vi "Create Test Class.vi"(8 "error in (no error)":errorcluster, 11 "Test Double Factory in":refnum<class "Test Double Factory.lvclass">) -> (0 "error out":errorcluster, 3 "Test Double Factory out":refnum<class "Test Double Factory.lvclass">)   [LabVIEW 2020, in "Test Double Factory.lvclass"]
uses:
  Test Double Factory.lvclass
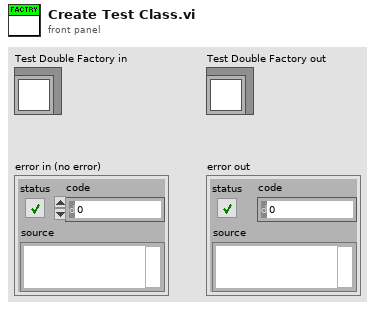
[diagram p1: front panel]
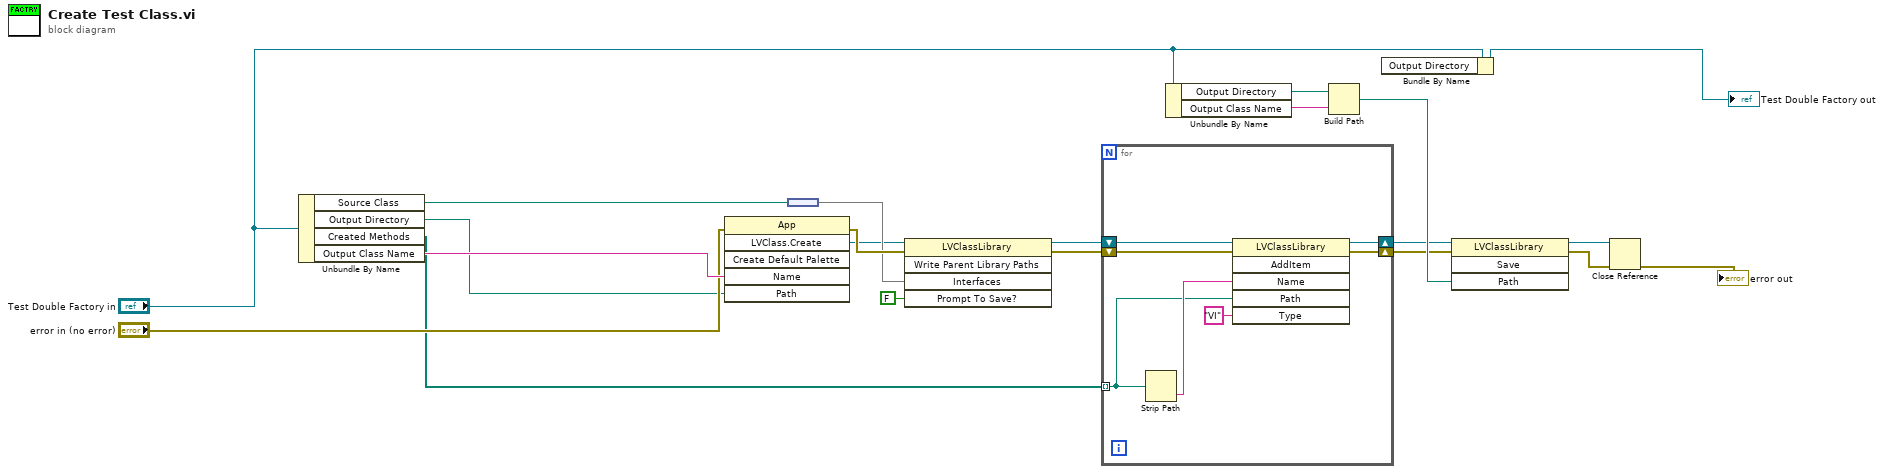
[diagram p0: block diagram]
diagram:
  n1 = Unbundle By Name("Test Double Factory in") -> ("Source Class"=w6:path, "Output Directory"=w5:path, "Created Methods"=w9:path[], "Output Class Name"=w19:string)
  n2 = invoke class="App" method="LVClass.Create"(error in="error in (no error)", "Name"=w19, "Path"=w5) -> (error out=w3:errorcluster, "LVClass.Create"=w1:refnum<vi>)  [unwired: 3 in, 4 out]
  n3 = node(w6) -> (w2:set{path})
  n4 = invoke class="LVClassLibrary" method="Write Parent Library Paths"(reference=w1, error in=w3, "Interfaces"=w2, "Prompt To Save?"=FALSE) -> (reference out=w4:refnum<vi>, error out=w8:errorcluster)  [unwired: 1 in, 3 out]
  n5 = for {
    shift-right: [w22] -> w12
    shift-left: w8 -> [w27]
    tunnel: w9 -> [w23] mode=indexing
    shift-right: [w24] -> w11
    shift-left: w4 -> [w28]
    n6 = Strip Path(path=w23) -> (name=w26:string)  [unwired: 1 out]
    n7 = invoke class="LVClassLibrary" method="AddItem"(reference=w28, error in=w27, "Name"=w26, "Path"=w23, "Type"="VI") -> (reference out=w24:refnum<vi>, error out=w22:errorcluster)  [unwired: 1 in, 4 out]
  }
  n8 = Unbundle By Name("Test Double Factory in") -> ("Output Directory"=w13:path, "Output Class Name"=w20:string)
  n9 = Build Path(base path=w13, name or relative path=w20) -> (appended path=w14:path)
  n10 = Bundle By Name(cluster="Test Double Factory in") -> (→"Test Double Factory out":refnum<class "Test Double Factory.lvclass">)  [unwired: 1 in]
  n11 = invoke class="LVClassLibrary" method="Save"(reference=w11, error in=w12, "Path"=w14) -> (reference out=w16:refnum<vi>, error out=w10:errorcluster)  [unwired: 1 in, 2 out]
  n12 = Close Reference(reference=w16, error in (no error)=w10) -> (error out=→"error out":errorcluster)
